vi "参数读写.vi"() -> ()   [LabVIEW 2016, in "超标留样集成.lvlib" / "德润DR803M超标留样.lvlib"]
uses:
  <vilib>/Utility/miscctls.llb/LVPointTypeDef.ctl
panel:
  in  "工作模式":u16(ring) items=["定时留样"=1, "时间等比"=2, "同步留样"=3, "外控留样"=4, "超标留样"=5]
  out "读取更新":bool
  in  "返回":bool
  in  "每瓶次数：":dbl
  in  "平行样：":dbl
  in  "每次留样：":dbl
  in  "留样瓶数：":dbl
  in  "当前瓶号：":dbl
  # "mL"
  # "mg/L"
  # "COD\n模拟\n设置"
  # "mg/L"
  # "mg/L"
  # "mg/L"
  # "mg/L"
  # "氨氮\n模拟\n设置"
  # "mg/L"
  # "mg/L"
  # "mg/L"
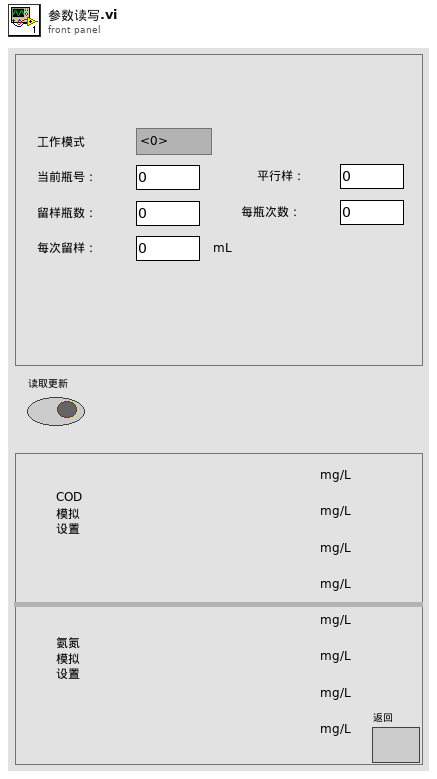
[diagram p1: front panel]
types:
  T1 = typedef "LVPointTypeDef.ctl" = cluster{"Horizontal":i16, "Vertical":i16}
  T2 = typedef "超标留样集成.lvlib/德润DR803M超标留样.lvlib/typedef.ctl" = cluster{"枚举":enum16{"open", "read", "write", "close", "write_register"}, "写入内容":string, "data_in":cluster{"write_coil_in":cluster{"address":u16, "value":bool}, "write_register_in":cluster{"address":u16, "values":u16[]}, "read_register_in":cluster{"starting address":u16, "quantity":u16}}}
  T3 = cluster{"采样器状态":enum16{"停止", "运行", "系统初始化-2", "系统初始化-3", "初始化失败"}, "仪器时间":timestamp, "留样结果":bool, "工作模式":u16, "当前瓶号":u16, "平行样数":u16, "采样瓶数":u16, "设定每瓶采样次数":u16, "每瓶采样量":u16, "当前进程":u16, "当前瓶已采次数":u16, "留样中":bool}
  T4 = cluster{"write_coil_in":cluster{"address":u16, "value":bool}, "write_register_in":cluster{"address":u16, "values":u16[]}, "read_register_in":cluster{"starting address":u16, "quantity":u16}}
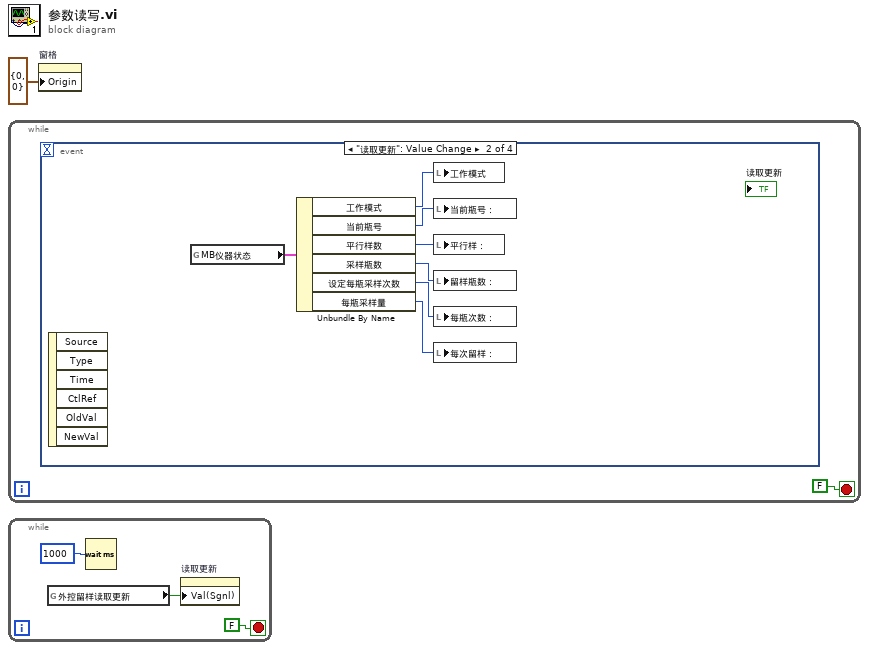
[diagram p0: block diagram]
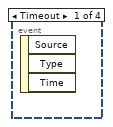
[diagram p2: hidden frame]
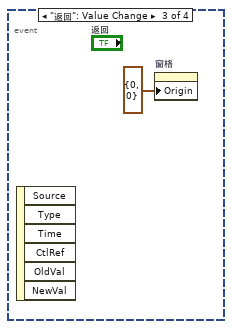
[diagram p3: hidden frame]
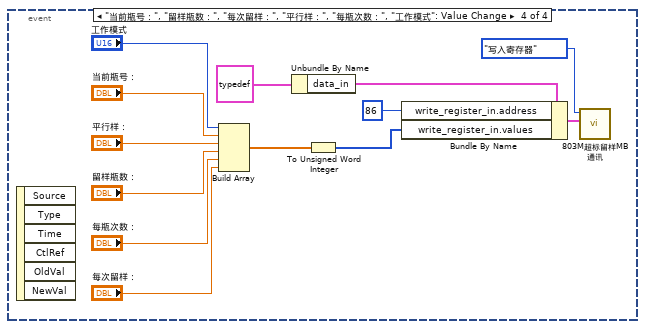
[diagram p4: hidden frame]
diagram:
  n1 = while {
    stop <- FALSE stop-if-true
    n2 = event shown="[1] \"读取更新\": Value Change" {
      selector: _ -> [_ _ _ _]
      dyn-events: _ -> [_ _ _ _]
      timeout: _ -> [_ _ _ _]
      event Timeout {
        n3 = event-data() -> ()  [unwired: 1 in, 3 out]
      }
      event "读取更新": Value Change {
        n4 = event-data() -> ()  [unwired: 1 in, 6 out]
        n5 = global read "超标留样全局.vi" "MB仪器状态"() -> (w9:T3)
        n6 = Unbundle By Name(w9) -> ("工作模式"=w3:u16, "当前瓶号"=w8:u16, "平行样数"=w7:u16, "采样瓶数"=w6:u16, "设定每瓶采样次数"=w5:u16, "每瓶采样量"=w4:u16)
        n7 = local write "工作模式"(w3) -> ()
        n8 = local write "当前瓶号："(w8) -> ()
        n9 = local write "平行样："(w7) -> ()
        n10 = local write "留样瓶数："(w6) -> ()
        n11 = local write "每瓶次数："(w5) -> ()
        n12 = local write "每次留样："(w4) -> ()
      }
      event "返回": Value Change {
        n13 = event-data() -> ()  [unwired: 1 in, 6 out]
        n14 = property on="窗格" class="Pane"("Origin"=T1 {"Horizontal"=0, "Vertical"=0} ("原点")) -> ()  [unwired: 2 in, 2 out]
      }
      event "当前瓶号：", "留样瓶数：", "每次留样：", "平行样：", "每瓶次数：", "工作模式": Value Change {
        n15 = event-data() -> ()  [unwired: 1 in, 6 out]
        n16 = Build Array("工作模式", "当前瓶号：", "平行样：", "留样瓶数：", "每瓶次数：", "每次留样：") -> (w12:dbl[])
        n17 = Unbundle By Name(T2 {"枚举"=enum."open", "写入内容"="超标留样", "data_in"={"write_coil_in"={"address"=0, "value"=FALSE}, "write_register_in"={"address"=0, "values"=[]}, "read_register_in"={"starting address"=0, "quantity"=0}}}) -> ("data_in"=w21:T4)
        n18 = To Unsigned Word Integer(number=w12) -> (unsigned 16bit integer=w11:u16[])
        n19 = Bundle By Name(cluster=w21, "write_register_in.address"=u16 86, "write_register_in.values"=w11) -> (w20:T4)
        n20 = call "803M超标留样MB通讯.vi"("data_in"=w20, "功能输入"=enum16{"打开串口", "写入", "读取", "关闭串口", "写入寄存器"}."写入寄存器") -> ()  [unwired: 8 in, 2 out]
      }
    }
  }
  n21 = while {
    stop <- FALSE stop-if-true
    n22 = global read "超标留样全局.vi" "外控留样读取更新"() -> (w24:bool)
    n23 = Wait (ms)(milliseconds to wait=u32 1000 ("等待时间（毫秒）")) -> ()  [unwired: 1 out]
    n24 = property on="读取更新" class="Bool (strict)"("Val(Sgnl)"=w24) -> ()  [unwired: 2 in, 2 out]
  }
  n25 = property on="窗格" class="Pane"("Origin"=T1 {"Horizontal"=0, "Vertical"=0} ("原点")) -> ()  [unwired: 2 in, 2 out]
